vi "Get Local Name and IP.vi"(0 "reset (F)":bool, 11 "error in":errorcluster) -> (4 "name":string, 6 "short name":string, 8 "IP address":string, 15 "error out":errorcluster)   [LabVIEW 2015, in "Car Wash.lvlib" / "AMC.lvlib"]
uses:
  AMC.lvlib
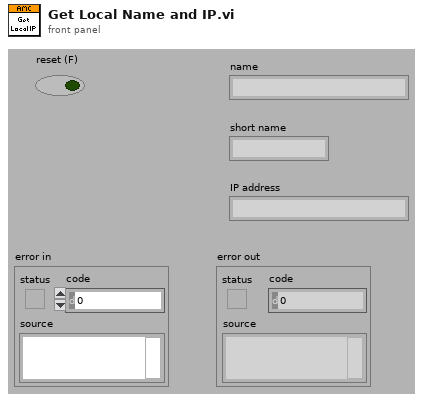
[diagram p1: front panel]
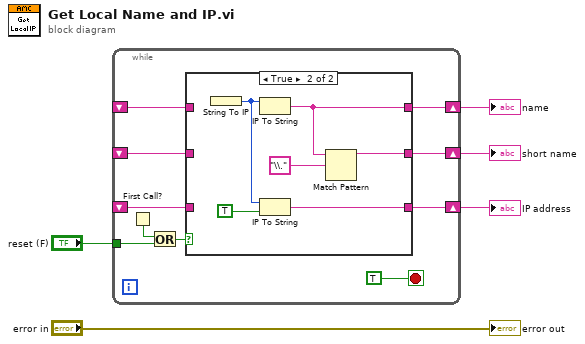
[diagram p0: block diagram]
diagram:
  n1 = while {
    shift-right: [w11] -> w5
    shift-left: _ -> [w9]
    shift-right: [w12] -> w4
    shift-left: _ -> [w8]
    shift-right: [w10] -> w3
    shift-left: _ -> [w7]
    tunnel: "reset (F)" -> [w6]
    stop <- TRUE stop-if-true
    n2 = First Call?() -> (First Call?: T/F=w14:bool)
    n3 = Or(x=w14, y=w6) -> (x .or. y?=w13:bool)
    n4 = case shown="True" w13 {
      tunnel: [w17 w21] -> w12
      tunnel: [w18 w20] -> w11
      tunnel: [w16 w19] -> w10
      tunnel: w9 -> [w18 _]
      tunnel: w8 -> [w17 _]
      tunnel: w7 -> [w16 _]
      frame False {
      }
      frame True {
        n5 = String To IP() -> (0:w23:u32)  [unwired: 1 out]
        n6 = IP To String(2:w23) -> (0:w20:string)  [unwired: 1 out]
        n7 = IP To String(1:TRUE ("dot notation? (F)"), 2:w23) -> (0:w19:string)
        n8 = Match Pattern(string=w20, regular expression="\\.") -> (before substring=w21:string)  [unwired: 4 out]
      }
    }
  }
  "name" <- w5
  "short name" <- w4
  "IP address" <- w3
  "error out" <- "error in"
